vi "Verify Config.vi"(8 "error in (no error)":errorcluster, 11 "Cfg Grandmaster in":refnum<class "Cfg Grandmaster.lvclass">) -> (0 "error out":errorcluster, 3 "Cfg Grandmaster out":refnum<class "Cfg Grandmaster.lvclass">)   [LabVIEW 2018, in "Configuration Grandmaster.lvlib" / "Cfg Grandmaster.lvclass"]
uses:
  Cfg Grandmaster.lvclass
  Cfg Grandmaster.lvclass/Cfg Grandmaster.ctl
  Data Acquisition/Class Chassis Tasks/Chassis Tasks.lvclass
  Class Chassis Cfg/ChassisCfg.lvclass
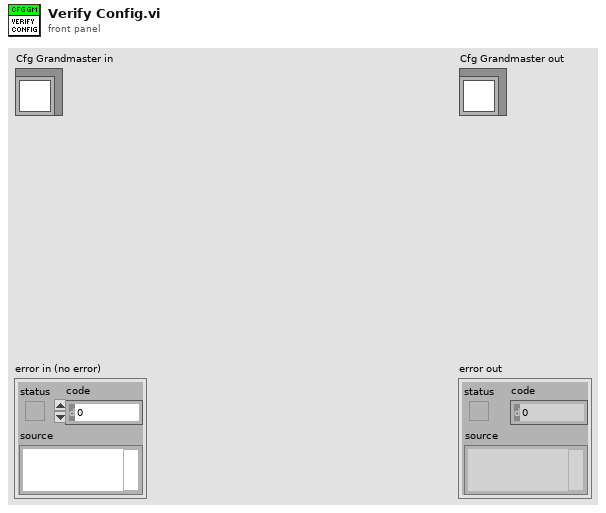
[diagram p1: front panel]
types:
  T1 = typedef "ge_Cfg wChassis.ctl" = cluster{"Chassis BOM":refnum<class "Chassis BOM.lvclass">, "Chassis Cfg":refnum<class "ChassisCfg.lvclass">, "Chassis Tasks":refnum<class "Chassis Tasks.lvclass">, "HW Error":bool, "Unsvd Chgs?":bool}
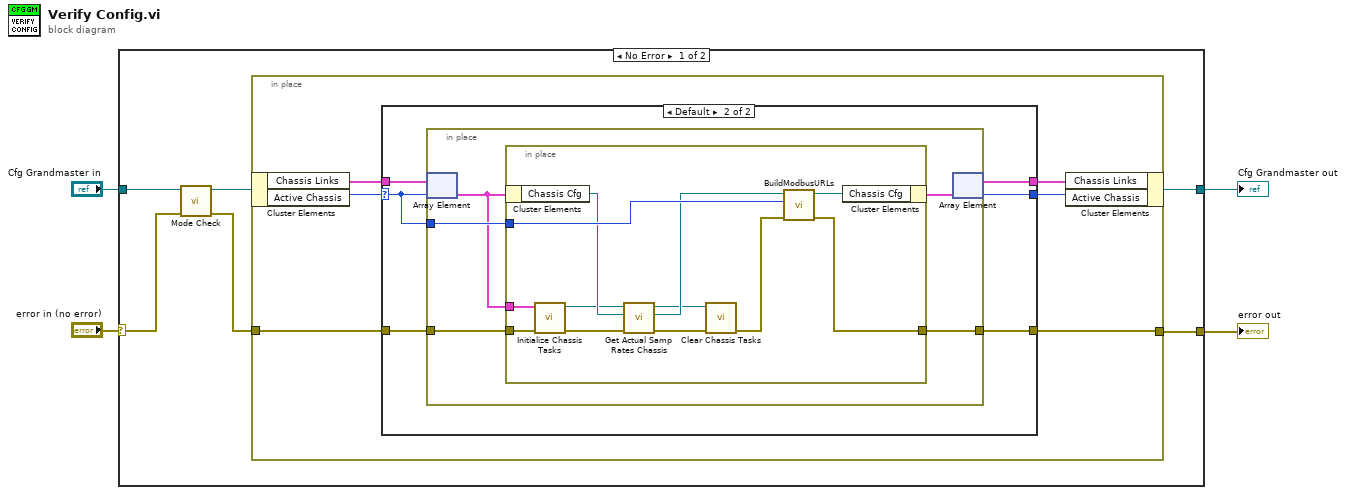
[diagram p0: block diagram]
diagram:
  n1 = case shown="No Error" "error in (no error)" {
    selector: "error in (no error)" -> [w8 w43]
    tunnel: [w7 w44] -> w2
    tunnel: "Cfg Grandmaster in" -> [w10 w44]
    tunnel: [w5 w43] -> w1
    frame No Error {
      n2 = call "Mode Check.vi"("error in (no error)"=w8, "Cfg Grandmaster in"=w10) -> ("error out"=w6:errorcluster, "Cfg Grandmaster out"=w9:refnum<class "Cfg Grandmaster.lvclass">)  [unwired: 8 in]
      n3 = in-place {
        in-place-border: w6 -> [w16]
        in-place-border: [w11] -> w5
        n4 = in-place-cluster #1(w9) -> ("Chassis Links"=w15:T1[], "Active Chassis"=w14:i32)
        n5 = case shown="Default" w14 {
          selector: w14 -> [w17 w21]
          tunnel: w15 -> [w19 w25]
          tunnel: [w19 w24] -> w13
          tunnel: w16 -> [w18 w23]
          tunnel: [w18 w22] -> w11
          tunnel: [w17 w20] -> w12
          frame -1 {
          }
          frame Default {
            n6 = in-place {
              in-place-border: w23 -> [w26]
              in-place-border: [w30] -> w22
              in-place-border: w21 -> [w29]
              n7 = in-place-array #2(w25, w21) -> (w27:T1)
              n8 = in-place {
                in-place-border: [w35] -> w30
                in-place-border: w29 -> [w42]
                in-place-border: w27 -> [w34]
                in-place-border: w26 -> [w32]
                n9 = in-place-cluster #3(w27) -> ("Chassis Cfg"=w40:refnum<class "ChassisCfg.lvclass">)
                n10 = call "Initialize Chassis Tasks.vi"("error in"=w32, "Cfg wChassis"=w34) -> ("error out"=w31:errorcluster, "Chassis Tasks out"=w33:refnum<class "Chassis Tasks.lvclass">)  [unwired: 8 in]
                n11 = call "Get Actual Samp Rates Chassis.vi"("error in (no error)"=w31, "Chassis Cfg"=w40, "Chassis Tasks in"=w33) -> ("error out"=w37:errorcluster, "Chassis Cfg"=w39:refnum<class "ChassisCfg.lvclass">, "Chassis Tasks out"=w38:refnum<class "Chassis Tasks.lvclass">)  [unwired: 6 in]
                n12 = call "Clear Chassis Tasks.vi"("error in (no error)"=w37, "Chassis Tasks in"=w38) -> ("error out"=w36:errorcluster)  [unwired: 8 in, 1 out]
                n13 = call "BuildModbusURLs.vi"("error in"=w36, "Chassis Num"=w42, "Chassis Cfg"=w39) -> ("error out"=w35:errorcluster, "Chassis Cfg"=w41:refnum<class "ChassisCfg.lvclass">)  [unwired: 7 in]
                n14 = in-place-cluster #3("Chassis Cfg"=w41) -> (w28:T1)
              }
              n15 = in-place-array #2(w28) -> (w24:T1[], w20:i32)
            }
          }
        }
        n16 = in-place-cluster #1("Chassis Links"=w13, "Active Chassis"=w12) -> (w7:refnum<class "Cfg Grandmaster.lvclass">)
      }
    }
    frame Error {
    }
  }
  "error out" <- w1
  "Cfg Grandmaster out" <- w2
